vi "Get IP String.vi"(0 "Display State In":T1={"Front Color"=1985280, "BkColor"=13816530} caption="显示状态输入", 5 "Front Color":u32(colorbox), 9 "Container State":T2 caption="容器状态", 11 "error in (no error)":errorcluster caption="错误输入（无错误）") -> (4 "Display State Out":T1={"Front Color"=1985280, "BkColor"=13816530} caption="显示状态输出", 15 "error out":errorcluster caption="错误输出")   [LabVIEW 2012, in "IP Adresss Control.xctl"]
uses:
  IP Adresss Control.xctl
  <vilib>/_xctls/Container State.ctl
  Core/IP Address Status.ctl
  <vilib>/_xctls/XControlSupport.lvlib
panel:
  # "添加构成方法参数的输入控件及显示控件。连接至连线板。不要删除已连接至连线板的输入控件及显示控件。\n\n如需设置该方法的参数，右键单击项目树中的对应项并选择“配置方法...”."
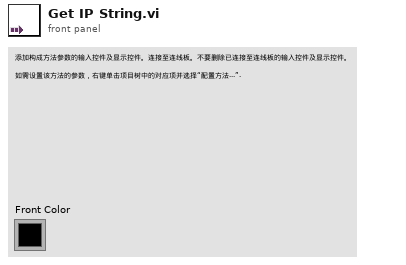
[diagram p1: front panel]
types:
  T1 = typedef "IP Adresss Control.xctl/IP Address Status.ctl" = cluster{"Front Color":u32, "BkColor":u32}
  T2 = typedef "XControlSupport.lvlib/Container State.ctl" = cluster{"Indicator?":bool, "Run Mode?":bool, " Refnum":refnum<vi>}
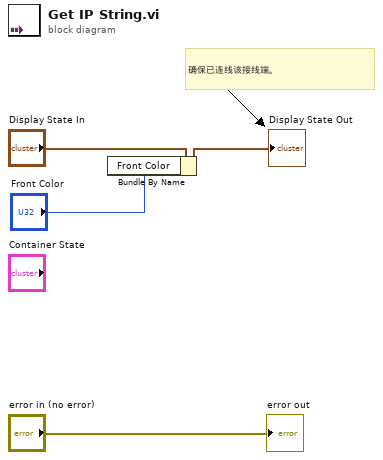
[diagram p0: block diagram]
diagram:
  # "确保已连线该接线端。"
  n1 = Bundle By Name(cluster="Display State In", "Front Color"="Front Color") -> (→"Display State Out":T1)
  "error out" <- "error in (no error)"
